vi "Variable Test.vi"() -> ()   [LabVIEW 2020, in "Library Core.lvlib" / "Sequencer (Default).lvclass"]
uses:
  Sequencer (Default).lvclass
panel:
  in  "Ref_Sequencer":refnum<vi>
  in  "Class Sequencer":refnum<class "Sequencer (Default).lvclass">
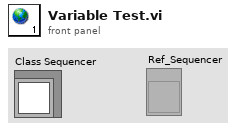
[diagram p1: front panel]
diagram:
